vi "Convert from MessagePackT format byte.vi"(8 "error in (no error)":errorcluster, 11 "Bytes in":u8[](array[numeric]) format="%x") -> (0 "error out":errorcluster, 1 "MsgPack Type":T2=enum."NEGINT", 2 "Object Family Type":T1, 3 "Bytes out":u8[](array[numeric]) format="%x")   [LabVIEW 2020, in "MessagePack.lvlib" / "MessagePack.lvclass"]
uses:
  MessagePack.lvclass
  IMessagePackObject/MsgPack Object Types.ctl
  Object Family.ctl
  <vilib>/Utility/error.llb/Error Cluster From Error Code.vi
  <vilib>/ErrorRing/Error Ring.xnode
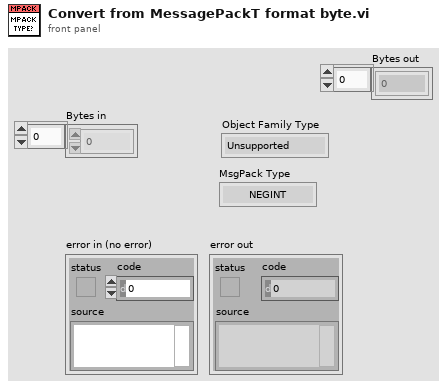
[diagram p1: front panel]
types:
  T1 = typedef "MessagePack.lvlib/MessagePack.lvclass/Object Family.ctl" = enum16{"Unsupported", "Nil", "Numeric", "Array", "Map", "String", "Binary", "Boolean", "Ext"}
  T2 = typedef "MessagePack.lvlib/MessagePack.lvclass/MsgPack Object Types.ctl" = enum16{"UNSUPPORTED", "POSINT", "NEGINT", "FIXMAP", "FIXARRAY", "FIXSTR", "NIL", "FALSE", "TRUE", "BIN8", "BIN16", "BIN32", "EXT8", "EXT16", "EXT32", "FLOAT32", "FLOAT64", "UINT8", "UINT16", "UINT32", "UINT64", "INT8", "INT16", "INT32", "INT64", "FIXEXT1", "FIXEXT2", "FIXEXT4", "FIXEXT8", "FIXEXT16", "STR8", "STR16", "STR32", "ARRAY16", "ARRAY32", "MAP16", "MAP32"}
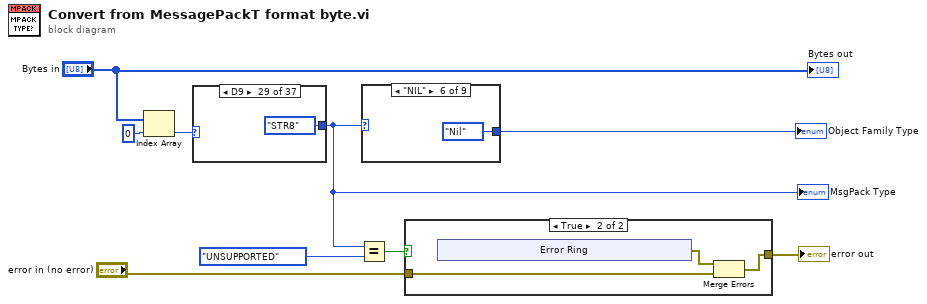
[diagram p0: block diagram]
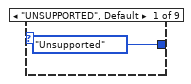
[diagram p2: hidden frame]
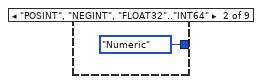
[diagram p3: hidden frame]
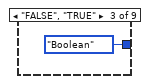
[diagram p4: hidden frame]
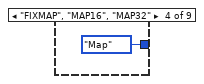
[diagram p5: hidden frame]
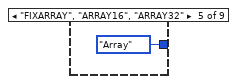
[diagram p6: hidden frame]
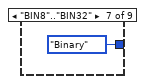
[diagram p7: hidden frame]
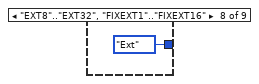
[diagram p8: hidden frame]
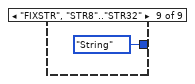
[diagram p9: hidden frame]
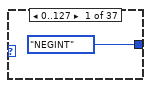
[diagram p11: hidden frame]
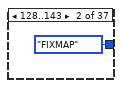
[diagram p12: hidden frame]
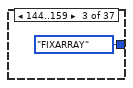
[diagram p13: hidden frame]
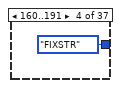
[diagram p14: hidden frame]
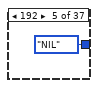
[diagram p15: hidden frame]
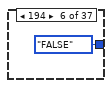
[diagram p16: hidden frame]
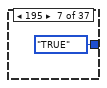
[diagram p17: hidden frame]
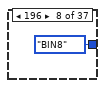
[diagram p18: hidden frame]
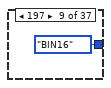
[diagram p19: hidden frame]
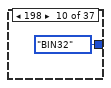
[diagram p20: hidden frame]
diagram:
  n1 = Index Array(array="Bytes in", index=0) -> (element=w3:u8)
  n2 = case shown="D9" w3 {
    tunnel: [MsgPack_Object_Types."NEGINT" ("Enum") MsgPack_Object_Types."FIXMAP" ("Enum") MsgPack_Object_Types."FIXARRAY" ("Enum") MsgPack_Object_Types."FIXSTR" ("Enum") MsgPack_Object_Types."NIL" ("Enum") MsgPack_Object_Types."FALSE" ("Enum") MsgPack_Object_Types."TRUE" ("Enum") MsgPack_Object_Types."BIN8" ("Enum") MsgPack_Object_Types."BIN16" ("Enum") MsgPack_Object_Types."BIN32" ("Enum") MsgPack_Object_Types."EXT8" ("Enum") MsgPack_Object_Types."EXT16" ("Enum") MsgPack_Object_Types."BIN32" ("Enum") MsgPack_Object_Types."FLOAT32" ("Enum") MsgPack_Object_Types."FLOAT64" ("Enum") MsgPack_Object_Types."UINT8" ("Enum") MsgPack_Object_Types."UINT16" ("Enum") MsgPack_Object_Types."UINT32" ("Enum") MsgPack_Object_Types."UINT64" ("Enum") MsgPack_Object_Types."INT8" ("Enum") MsgPack_Object_Types."INT16" ("Enum") MsgPack_Object_Types."INT32" ("Enum") MsgPack_Object_Types."INT64" ("Enum") MsgPack_Object_Types."FIXEXT1" ("Enum") MsgPack_Object_Types."FIXEXT2" ("Enum") MsgPack_Object_Types."FIXEXT4" ("Enum") MsgPack_Object_Types."FIXEXT8" ("Enum") MsgPack_Object_Types."FIXEXT16" ("Enum") MsgPack_Object_Types."STR8" ("Enum") MsgPack_Object_Types."STR16" ("Enum") MsgPack_Object_Types."STR32" ("Enum") MsgPack_Object_Types."ARRAY16" ("Enum") MsgPack_Object_Types."ARRAY32" ("Enum") MsgPack_Object_Types."MAP16" ("Enum") MsgPack_Object_Types."MAP32" ("Enum") MsgPack_Object_Types."UNSUPPORTED" ("Enum") MsgPack_Object_Types."NEGINT" ("Enum")] -> w2
    frame 0..127 {
    }
    frame 128..143 {
    }
    frame 144..159 {
    }
    frame 160..191 {
    }
    frame 192 {
    }
    frame 194 {
    }
    frame 195 {
    }
    frame 196 {
    }
    frame 197 {
    }
    frame 198 {
    }
    frame 199 {
    }
    frame 200 {
    }
    frame 201 {
    }
    frame 202 {
    }
    frame 203 {
    }
    frame 204 {
    }
    frame 205 {
    }
    frame 206 {
    }
    frame 207 {
    }
    frame 208 {
    }
    frame 209 {
    }
    frame 210 {
    }
    frame 211 {
    }
    frame 212 {
    }
    frame 213 {
    }
    frame 214 {
    }
    frame 215 {
    }
    frame 216 {
    }
    frame 217 {
    }
    frame 218 {
    }
    frame 219 {
    }
    frame 220 {
    }
    frame 221 {
    }
    frame 222 {
    }
    frame 223 {
    }
    frame Default {
    }
    frame 224..255 {
    }
  }
  "MsgPack Type" <- w2
  n3 = Equal?(x=w2, y=MsgPack_Object_Types."UNSUPPORTED") -> (x = y?=w7:bool)
  n4 = case shown="\"NIL\"" w2 {
    tunnel: [Object_Family."Unsupported" ("Object Family") Object_Family."Numeric" ("Object Family") Object_Family."Boolean" ("Object Family") Object_Family."Map" ("Object Family") Object_Family."Array" ("Object Family") Object_Family."Nil" ("Object Family") Object_Family."Binary" ("Object Family") Object_Family."Ext" ("Object Family") Object_Family."String" ("Object Family")] -> w1
    frame "UNSUPPORTED", Default {
    }
    frame "POSINT", "NEGINT", "FLOAT32".."INT64" {
    }
    frame "FALSE", "TRUE" {
    }
    frame "FIXMAP", "MAP16", "MAP32" {
    }
    frame "FIXARRAY", "ARRAY16", "ARRAY32" {
    }
    frame "NIL" {
    }
    frame "BIN8".."BIN32" {
    }
    frame "EXT8".."EXT32", "FIXEXT1".."FIXEXT16" {
    }
    frame "FIXSTR", "STR8".."STR32" {
    }
  }
  "Object Family Type" <- w1
  n5 = case shown="True" w7 {
    tunnel: "error in (no error)" -> [w56 w58]
    tunnel: [w56 w57] -> w6
    frame False {
    }
    frame True {
      n6 = xnode "Error Ring"() -> ("error out"=w59:errorcluster)
      n7 = Merge Errors(w59, w58) -> (w57:errorcluster)
    }
  }
  "error out" <- w6
  "Bytes out" <- "Bytes in"
